vi "Timer Tester.vi"() -> ()   [LabVIEW 2010]
doc: "This VI is a quick tester for the Timer with Pause VI. It is not part of the delivered application."
uses:
  Controls/Timer Actions ENUM_TEST_TDef.ctl
panel:
  in  "OK Button":bool
  in  "Timer Action":T1
  in  "Target Time":dbl
  out "Elapsed Time":dbl format="%.2g"
  out "Done?":bool
  in  "stop":bool
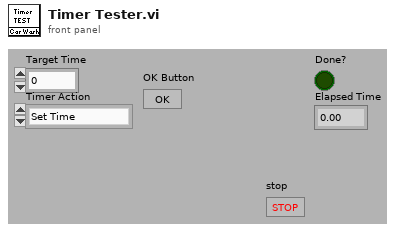
[diagram p1: front panel]
types:
  T1 = typedef "Timer Actions ENUM_TEST_TDef.ctl" = enum16{"Set Time", "Get Time", "Pause Time", "Resume Time"}
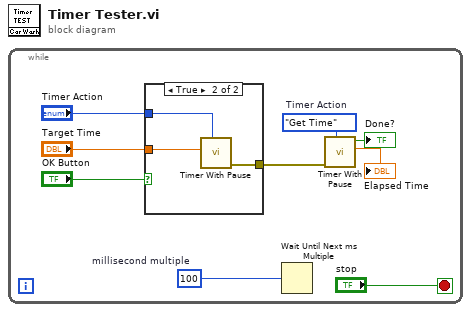
[diagram p0: block diagram]
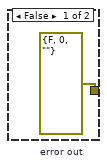
[diagram p2: hidden frame]
diagram:
  n1 = while {
    stop <- "stop" stop-if-true
    w7 = Timer_Actions_ENUM_TEST_TDef."Get Time"  # Timer Action
    w8 = u32 100  # millisecond multiple
    n2 = case shown="True" "OK Button" {
      tunnel: [w10 w13] -> w4
      tunnel: "Target Time" -> [_ w12]
      tunnel: "Timer Action" -> [_ w11]
      frame False {
        w10 = errorcluster {"status"=FALSE, "code"=0, "source"=""}  # error out
      }
      frame True {
        n3 = call "Timer With Pause.vi"("Timer Action"=w11, "Target Time"=w12) -> ("error out"=w13:errorcluster)  [unwired: 6 in, 3 out]
      }
    }
    n4 = Wait Until Next ms Multiple(millisecond multiple=w8) -> ()  [unwired: 1 out]
    n5 = call "Timer With Pause.vi"("Timer Action"=w7, "error in (no error)"=w4) -> ("Elapsed Time"=→"Elapsed Time":dbl, "Done?"=→"Done?":bool)  [unwired: 6 in, 2 out]
  }
